vi "Get Coil Constant.vi"(2 "error in":T2, 3 "Communications Config":T1={"GPIB address"=22, "GPIB bus"=0, "connection ID"=refnum, "IP"="192.168.2.200", "Active Comm Interface"=0, "Serial Port"="", "Programmer Type"=0} {"Programmer Type" items=["Model 430", "Model 420"]; "Active Comm Interface" items=["TCP/IP (Model 430 Only)", "RS232", "IEEE488"]}) -> (0 "error out":T2, 1 "Coil Constant":dbl format="%.3f")   [LabVIEW 2019]
panel:
  in  "GPIB Address":cluster{"GPIB address":i16, "GPIB bus":i16}={"GPIB address"=22, "GPIB bus"=0}
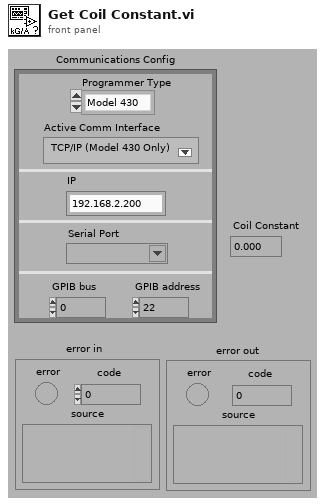
[diagram p1: front panel]
types:
  T1 = cluster{"GPIB address":i16, "GPIB bus":i16, "connection ID":refnum<k5>, "IP":string, "Active Comm Interface":u16, "Serial Port":refnum<visa-resource-name>, "Programmer Type":u16}
  T2 = cluster{"error":bool, "code":i32, "source":string}
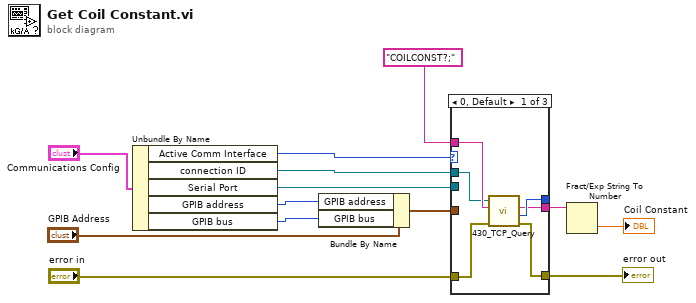
[diagram p0: block diagram]
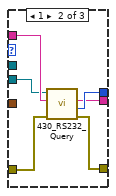
[diagram p2: hidden frame]
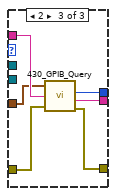
[diagram p3: hidden frame]
diagram:
  n1 = Unbundle By Name("Communications Config") -> ("Active Comm Interface"=w8:u16, "connection ID"=w7:refnum<k5>, "Serial Port"=w9:refnum<visa-resource-name>, "GPIB address"=w11:i16, "GPIB bus"=w12:i16)
  n2 = Bundle By Name(cluster="GPIB Address", "GPIB address"=w11, "GPIB bus"=w12) -> (w6:cluster{"GPIB address":i16, "GPIB bus":i16})
  n3 = case shown="0, Default" w8 {
    tunnel: "COILCONST?;" -> [w18 w24 w31]
    tunnel: "error in" -> [w14 w20 w30]
    tunnel: [w19 w25 w29] -> w2
    tunnel: [w16 w22 w27] -> w3
    tunnel: [w17 w23 w28] -> _
    tunnel: w9 -> [_ w21 _]
    tunnel: w7 -> [w15 _ _]
    tunnel: w6 -> [_ _ w26]
    frame 0, Default {
      n4 = call "430_TCP_Query.vi"("error in (no error)"=w14, "Command"=w18, "connection ID"=w15) -> ("error out"=w19:errorcluster, "Bytes Read"=w17:i32, "Response"=w16:string)  [unwired: 4 in, 2 out]
    }
    frame 1 {
      n5 = call "430_RS232_Query.vi"("error in (no error)"=w20, "Command"=w24, "VISA resource name"=w21) -> ("error out"=w25:errorcluster, "Bytes Read"=w23:i32, "Response"=w22:string)  [unwired: 4 in, 2 out]
    }
    frame 2 {
      n6 = call "430_GPIB_Query.vi"("GPIB (In)"=w26, "Input query"=w31, "error in"=w30) -> ("Bytes returned"=w28:i32, "Return string"=w27:string, "error out"=w29:T2)  [unwired: 1 out]
    }
  }
  "error out" <- w2
  n7 = Fract/Exp String To Number(string=w3) -> (number=→"Coil Constant":dbl)  [unwired: 3 in, 1 out]
